vi "Frame.Settings.vi"(6 "Action":enum8{"Get", "Set"}(ring), 8 "error in (no error)":errorcluster, 10 "Frame.Settings":T1={"ID"=0, "Disable Transmission"=FALSE, "Disable Transmission Ref"=18446744073709551615, "Transmit Trigger"=enum."Channel value change", "Transmit Trigger Ref"=18446744073709551615} {"Transmit Trigger Ref" format="%.0x"; "Disable Transmission Ref" format="%.0x"}, 11 "Item Ref in":T2 format="%.0x") -> (0 "error out":errorcluster, 2 "Frame.Settings":T1={"ID"=0, "Disable Transmission"=FALSE, "Disable Transmission Ref"=18446744073709551615, "Transmit Trigger"=enum."Channel value change", "Transmit Trigger Ref"=18446744073709551615} {"Transmit Trigger Ref" format="%.0x"; "Disable Transmission Ref" format="%.0x"}, 3 "Item Ref out":T2 format="%.0x")   [LabVIEW 2019, in "Protection and Counter Addon System Explorer.lvlib"]
uses:
  Protection and Counter Addon System Explorer.lvlib
  <vilib>/NI VeriStand/Custom Device API/Custom Device Item Ref.ctl
  Types/Frame Settings.ctl
  Types/Event Trigger Type.ctl
  Addon Shared/SubVIs/GUID Lookup.vi
  <vilib>/NI VeriStand/Custom Device API/Set Item Property (Dependent Node Pointer).vi
  <vilib>/NI VeriStand/Custom Device API/Set Item Property (U32).vi
  <vilib>/NI VeriStand/Custom Device API/Set Item Property (Boolean).vi
  <vilib>/NI VeriStand/Custom Device API/Get Item Property (Dependent Node Pointer).vi
  <vilib>/NI VeriStand/Custom Device API/Get Item Property (U32).vi
  <vilib>/NI VeriStand/Custom Device API/Get Item Property (Boolean).vi
  <vilib>/NI VeriStand/Custom Device API/Custom Device API.lvlib
  Addon Shared/Protection and Counter Addon Shared.lvlib
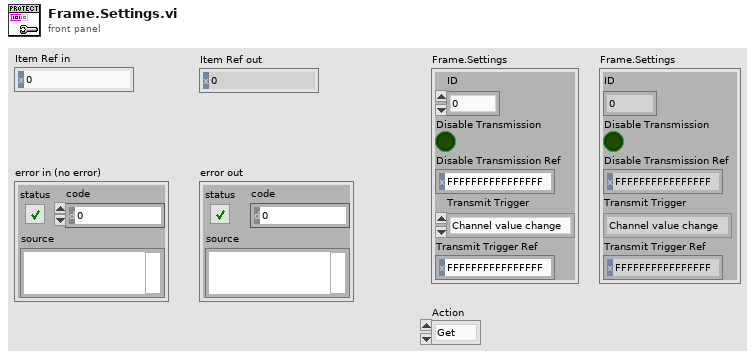
[diagram p1: front panel]
types:
  T1 = typedef "Protection and Counter Addon System Explorer.lvlib/Frame Settings.ctl" = cluster{"ID":u32, "Disable Transmission":bool, "Disable Transmission Ref":T2, "Transmit Trigger":T3, "Transmit Trigger Ref":T2}
  T2 = typedef "Custom Device API.lvlib/Custom Device Item Ref.ctl" = u64
  T3 = typedef "Protection and Counter Addon System Explorer.lvlib/Event Trigger Type.ctl" = enum16{"Channel value change", "Trigger channel (not zero)", "Channel value change or trigger channel (not zero)", "Trigger channel (any value change)", "Channel value change or trigger channel (any value change)"}
  T4 = typedef "Custom Device API.lvlib/Custom Device Item Info.ctl" = cluster{"Name":string, "Is Channel":bool, "GUID":string, "Is Waveform":bool}
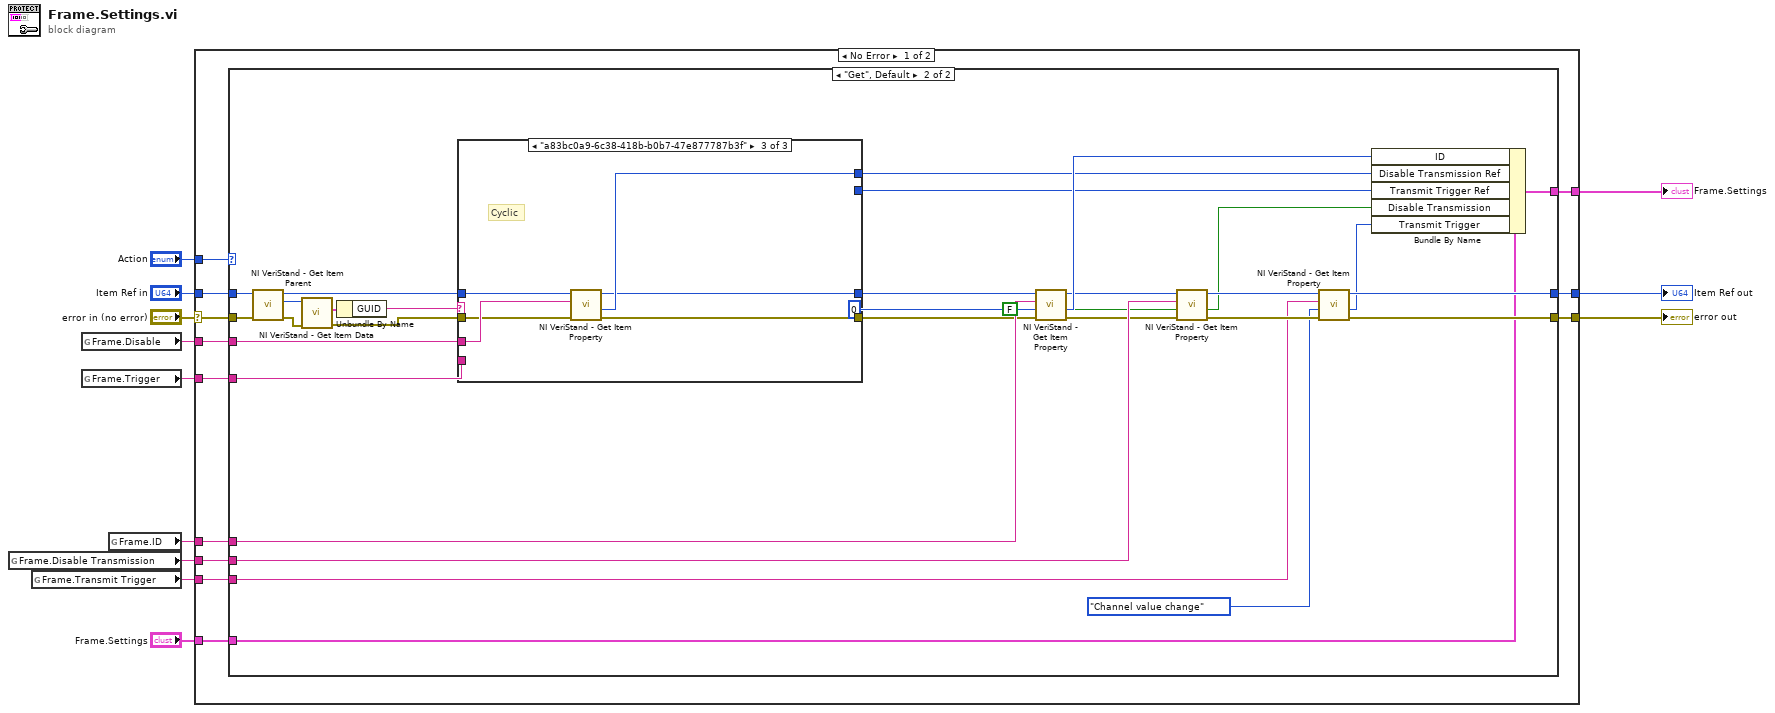
[diagram p0: block diagram]
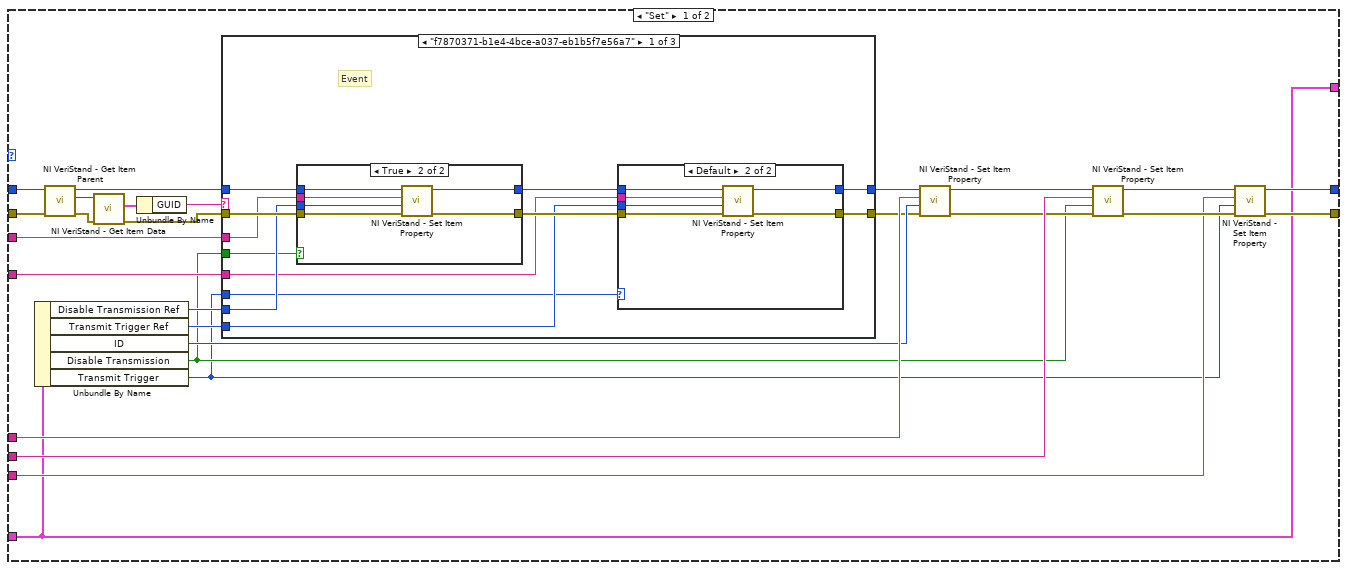
[diagram p2: hidden frame]
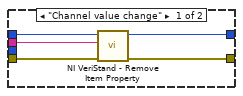
[diagram p3: hidden frame]
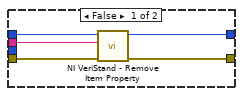
[diagram p4: hidden frame]
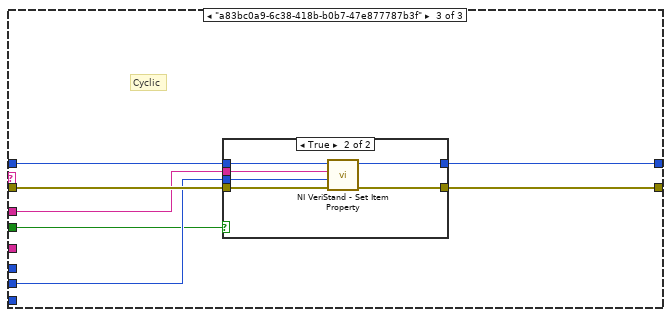
[diagram p6: hidden frame]
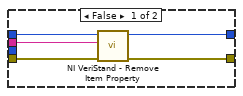
[diagram p7: hidden frame]
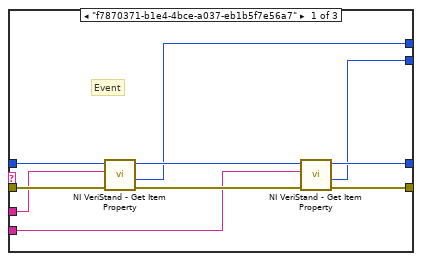
[diagram p8: hidden frame]
diagram:
  n1 = global read "GUID Lookup.vi" "Frame.Disable Transmission"() -> (w4:string)
  n2 = global read "GUID Lookup.vi" "Frame.Transmit Trigger"() -> (w5:string)
  n3 = global read "GUID Lookup.vi" "Frame.Disable"() -> (w1:string)
  n4 = global read "GUID Lookup.vi" "Frame.Trigger"() -> (w2:string)
  n5 = global read "GUID Lookup.vi" "Frame.ID"() -> (w3:string)
  n6 = case shown="No Error" "error in (no error)" {
    selector: "error in (no error)" -> [w15 w155]
    tunnel: "Item Ref in" -> [w24 w154]
    tunnel: w3 -> [w23 _]
    tunnel: w1 -> [w22 _]
    tunnel: w2 -> [w21 _]
    tunnel: [w20 w155] -> w11
    tunnel: [w19 w154] -> w10
    tunnel: [w18 _] -> w9
    tunnel: w5 -> [w17 _]
    tunnel: w4 -> [w16 _]
    tunnel: "Frame.Settings" -> [w14 _]
    tunnel: "Action" -> [w13 _]
    frame No Error {
      n7 = case shown="\"Get\", Default" w13 {
        tunnel: w24 -> [w37 w115]
        tunnel: w23 -> [w50 w135]
        tunnel: w22 -> [w34 w110]
        tunnel: w21 -> [w33 w109]
        tunnel: [w47 w131] -> w20
        tunnel: [w46 w130] -> w19
        tunnel: [w43 w123] -> w18
        tunnel: w17 -> [w45 w129]
        tunnel: w16 -> [w44 w128]
        tunnel: w15 -> [w36 w112]
        tunnel: w14 -> [w43 w124]
        frame "Set" {
          n8 = Unbundle By Name(w43) -> ("Disable Transmission Ref"=w28:T2, "Transmit Trigger Ref"=w27:T2, "ID"=w42:u32, "Disable Transmission"=w26:bool, "Transmit Trigger"=w25:T3)
          n9 = call <vilib>:"NI VeriStand - Get Item Parent.vi"("error in (no error)"=w36, "Item Ref in"=w37) -> ("error out"=w32:errorcluster, "Parent Ref"=w39:T2, "Item Ref out"=w38:T2)  [unwired: 6 in, 1 out]
          n10 = call <vilib>:"NI VeriStand - Get Item Data.vi"("error in (no error)"=w32, "Item Ref in"=w39) -> ("error out"=w35:errorcluster, "Item Info"=w40:T4)  [unwired: 8 out]
          n11 = Unbundle By Name(w40) -> ("GUID"=w41:string)
          n12 = case shown="\"f7870371-b1e4-4bce-a037-eb1b5f7e56a7\"" w41 {
            tunnel: w35 -> [w62 w86 w93]
            tunnel: [w52 w86 w88] -> w31
            tunnel: w34 -> [w61 _ w91]
            tunnel: w33 -> [w55 _ _]
            tunnel: w38 -> [w60 w85 w90]
            tunnel: [w53 w85 w89] -> _
            tunnel: w28 -> [w59 _ w92]
            tunnel: w27 -> [w56 _ _]
            tunnel: w26 -> [w58 _ w87]
            tunnel: w25 -> [w51 _ _]
            frame "f7870371-b1e4-4bce-a037-eb1b5f7e56a7" {
              # "Event"
              n13 = case shown="True" w58 {
                tunnel: [w74 w84] -> w54
                tunnel: [w75 w83] -> w57
                tunnel: w62 -> [w76 w82]
                tunnel: w61 -> [w77 w81]
                tunnel: w60 -> [w78 w80]
                tunnel: w59 -> [_ w79]
                frame False {
                  n14 = call <vilib>:"NI VeriStand - Remove Item Property.vi"("error in (no error)"=w76, "Property Name"=w77, "Item Ref in"=w78) -> ("error out"=w75:errorcluster, "Item Ref out"=w74:T2)  [unwired: 6 in, 1 out]
                }
                frame True {
                  n15 = call-poly <vilib>:"NI VeriStand - Set Item Property.vi"("error in (no error)"=w82, "Dependent Node Ref"=w79, "Property Name"=w81, "Item Ref in"=w80) -> ("error out"=w83:errorcluster, "Item Ref out"=w84:T2)  [unwired: 5 in, 1 out]
                }
              }
              n16 = case shown="Default" w51 {
                tunnel: [w63 w73] -> w53
                tunnel: [w64 w72] -> w52
                tunnel: w57 -> [w65 w71]
                tunnel: w55 -> [w66 w70]
                tunnel: w54 -> [w67 w69]
                tunnel: w56 -> [_ w68]
                frame "Channel value change" {
                  n17 = call <vilib>:"NI VeriStand - Remove Item Property.vi"("error in (no error)"=w65, "Property Name"=w66, "Item Ref in"=w67) -> ("error out"=w64:errorcluster, "Item Ref out"=w63:T2)  [unwired: 6 in, 1 out]
                }
                frame Default {
                  n18 = call-poly <vilib>:"NI VeriStand - Set Item Property.vi"("error in (no error)"=w71, "Dependent Node Ref"=w68, "Property Name"=w70, "Item Ref in"=w69) -> ("error out"=w72:errorcluster, "Item Ref out"=w73:T2)  [unwired: 5 in, 1 out]
                }
              }
            }
            frame "45d997b9-be87-4536-8aa7-486032a53b20", Default {
              # "SinglePoint"
            }
            frame "a83bc0a9-6c38-418b-b0b7-47e877787b3f" {
              # "Cyclic"
              n19 = case shown="True" w87 {
                tunnel: [w94 w104] -> w89
                tunnel: [w95 w103] -> w88
                tunnel: w93 -> [w96 w102]
                tunnel: w91 -> [w97 w101]
                tunnel: w90 -> [w98 w100]
                tunnel: w92 -> [_ w99]
                frame False {
                  n20 = call <vilib>:"NI VeriStand - Remove Item Property.vi"("error in (no error)"=w96, "Property Name"=w97, "Item Ref in"=w98) -> ("error out"=w95:errorcluster, "Item Ref out"=w94:T2)  [unwired: 6 in, 1 out]
                }
                frame True {
                  n21 = call-poly <vilib>:"NI VeriStand - Set Item Property.vi"("error in (no error)"=w102, "Dependent Node Ref"=w99, "Property Name"=w101, "Item Ref in"=w100) -> ("error out"=w103:errorcluster, "Item Ref out"=w104:T2)  [unwired: 5 in, 1 out]
                }
              }
            }
          }
          n22 = call-poly <vilib>:"NI VeriStand - Set Item Property.vi"("error in (no error)"=w31, "Value"=w42, "Property Name"=w50, "Item Ref in"=w37) -> ("error out"=w30:errorcluster, "Item Ref out"=w29:T2)  [unwired: 5 in, 1 out]
          n23 = call-poly <vilib>:"NI VeriStand - Set Item Property.vi"("error in (no error)"=w30, "Value"=w26, "Property Name"=w44, "Item Ref in"=w29) -> ("error out"=w48:errorcluster, "Item Ref out"=w49:T2)  [unwired: 5 in, 1 out]
          n24 = call-poly <vilib>:"NI VeriStand - Set Item Property.vi"("error in (no error)"=w48, "Value"=w25, "Property Name"=w45, "Item Ref in"=w49) -> ("error out"=w47:errorcluster, "Item Ref out"=w46:T2)  [unwired: 5 in, 1 out]
        }
        frame "Get", Default {
          n25 = call <vilib>:"NI VeriStand - Get Item Parent.vi"("error in (no error)"=w112, "Item Ref in"=w115) -> ("error out"=w116:errorcluster, "Parent Ref"=w117:T2, "Item Ref out"=w108:T2)  [unwired: 6 in, 1 out]
          n26 = call <vilib>:"NI VeriStand - Get Item Data.vi"("error in (no error)"=w116, "Item Ref in"=w117) -> ("error out"=w118:errorcluster, "Item Info"=w119:T4)  [unwired: 8 out]
          n27 = Unbundle By Name(w119) -> ("GUID"=w120:string)
          n28 = case shown="\"a83bc0a9-6c38-418b-b0b7-47e877787b3f\"" w120 {
            tunnel: w118 -> [w143 w147 w151]
            tunnel: [w142 w147 w150] -> w111
            tunnel: w110 -> [w141 _ w153]
            tunnel: w109 -> [w140 _ _]
            tunnel: w108 -> [w139 w146 w152]
            tunnel: [w138 w146 w148] -> w107
            tunnel: [w137 _ w149] -> w106
            tunnel: [w136 _ _] -> w105
            frame "f7870371-b1e4-4bce-a037-eb1b5f7e56a7" {
              # "Event"
              n29 = call-poly <vilib>:"NI VeriStand - Get Item Property.vi"("error in (no error)"=w143, "Property Name"=w141, "Item Ref in"=w139) -> ("error out"=w144:errorcluster, "Dependent Node Ref"=w137:T2, "Item Ref out"=w145:T2)  [unwired: 5 in, 1 out]
              n30 = call-poly <vilib>:"NI VeriStand - Get Item Property.vi"("error in (no error)"=w144, "Property Name"=w140, "Item Ref in"=w145) -> ("error out"=w142:errorcluster, "Dependent Node Ref"=w136:T2, "Item Ref out"=w138:T2)  [unwired: 5 in, 1 out]
            }
            frame "45d997b9-be87-4536-8aa7-486032a53b20", Default {
              # "SinglePoint"
            }
            frame "a83bc0a9-6c38-418b-b0b7-47e877787b3f" {
              # "Cyclic"
              n31 = call-poly <vilib>:"NI VeriStand - Get Item Property.vi"("error in (no error)"=w151, "Property Name"=w153, "Item Ref in"=w152) -> ("error out"=w150:errorcluster, "Dependent Node Ref"=w149:T2, "Item Ref out"=w148:T2)  [unwired: 5 in, 1 out]
            }
          }
          n32 = call-poly <vilib>:"NI VeriStand - Get Item Property.vi"("error in (no error)"=w111, "Default Value"=u32 0, "Property Name"=w135, "Item Ref in"=w107) -> ("error out"=w114:errorcluster, "Value"=w127:u32, "Item Ref out"=w113:T2)  [unwired: 4 in, 1 out]
          n33 = call-poly <vilib>:"NI VeriStand - Get Item Property.vi"("error in (no error)"=w114, "Default Value"=FALSE, "Property Name"=w128, "Item Ref in"=w113) -> ("error out"=w132:errorcluster, "Value"=w125:bool, "Item Ref out"=w133:T2)  [unwired: 4 in, 1 out]
          n34 = call-poly <vilib>:"NI VeriStand - Get Item Property.vi"("error in (no error)"=w132, "Default Value"=Event_Trigger_Type."Channel value change" ("Transmit Trigger"), "Property Name"=w129, "Item Ref in"=w133) -> ("error out"=w131:errorcluster, "Value"=w126:u32, "Item Ref out"=w130:T2)  [unwired: 4 in, 1 out]
          n35 = Bundle By Name(cluster=w124, "ID"=w127, "Disable Transmission Ref"=w106, "Transmit Trigger Ref"=w105, "Disable Transmission"=w125, "Transmit Trigger"=w126) -> (w123:T1)
        }
      }
    }
    frame Error {
    }
  }
  "Item Ref out" <- w10
  "error out" <- w11
  "Frame.Settings" <- w9
